vi "CSTK_Button_Icon_Example.vi"() -> ()   [LabVIEW 2015]
uses:
  Library/Button Icon/CSTK_Button_Icon.xctl
  Library/Button Icon/Private/TypeDefinitions/CSTK_Button_Icon_Properties_Color.ctl
  Library/Button Icon/Private/TypeDefinitions/CSTK_Button_Icon_Properties_BorderWidth.ctl
  Library/Button Icon/Private/TypeDefinitions/CSTK_Button_Icon_Properties_BorderStyle.ctl
  Library/Button Icon/Private/TypeDefinitions/CSTK_Button_Icon_Properties_BorderRadius.ctl
  Library/Button Icon/Private/TypeDefinitions/CSTK_Button_Icon_Properties_BoolText.ctl
  Library/Button Icon/Private/TypeDefinitions/CSTK_Button_Icon_Properties_HorizontalOffset.ctl
  Library/Button Icon/Private/TypeDefinitions/CSTK_Button_Icon_Properties_Display.ctl
  Library/Button Icon/Private/TypeDefinitions/CSTK_Button_Icon_Properties_FontStyle.ctl
  Library/Button Icon/Private/TypeDefinitions/_CSTK_Button_Icon_TextProperties_FontStyle.ctl
panel:
  in  "LOGO:显示LOGO":T1
  in  "LOGO:水平偏移":T2
  in  "布尔文本:字体样式":T3={"False"={"Font Name"="", "Size"=17, "Strikeout?"=FALSE, "Italic?"=FALSE, "Underline?"=FALSE, "Outline?"=FALSE, "Shadow?"=FALSE, "Bold?"=FALSE}, "True"={"Font Name"="", "Size"=17, "Strikeout?"=FALSE, "Italic?"=FALSE, "Underline?"=FALSE, "Outline?"=FALSE, "Shadow?"=FALSE, "Bold?"=FALSE}, "True to False"={"Font Name"="", "Size"=17, "Strikeout?"=FALSE, "Italic?"=FALSE, "Underline?"=FALSE, "Outline?"=FALSE, "Shadow?"=FALSE, "Bold?"=FALSE}, "False to True"={"Font Name"="", "Size"=17, "Strikeout?"=FALSE, "Italic?"=FALSE, "Underline?"=FALSE, "Outline?"=FALSE, "Shadow?"=FALSE, "Bold?"=FALSE}, "Hover in False"={"Font Name"="", "Size"=17, "Strikeout?"=FALSE, "Italic?"=FALSE, "Underline?"=FALSE, "Outline?"=FALSE, "Shadow?"=FALSE, "Bold?"=FALSE}, "Hover in True"={"Font Name"="", "Size"=17, "Strikeout?"=FALSE, "Italic?"=FALSE, "Underline?"=FALSE, "Outline?"=FALSE, "Shadow?"=FALSE, "Bold?"=FALSE}}
  in  "布尔文本:显示文本":T1
  in  "布尔文本:文本颜色":T5
  in  "布尔文本:水平偏移":T2
  in  "布尔文本":T6
  in  "边框颜色":T5
  in  "边框属性:圆角半径":T7
  in  "边框属性:线条样式":T8
  in  "边框属性:线条宽度":T9
  in  "背景颜色":T5
  in  "按钮大小":cluster{"Width":u32, "Height":u32}
  in  "停止VI按钮":bool
  in  "写入属性":bool
  in  "刷新属性":bool
  in  "CSTK_Button_Icon_Control":bool(xcontrol)
  out "Record":string
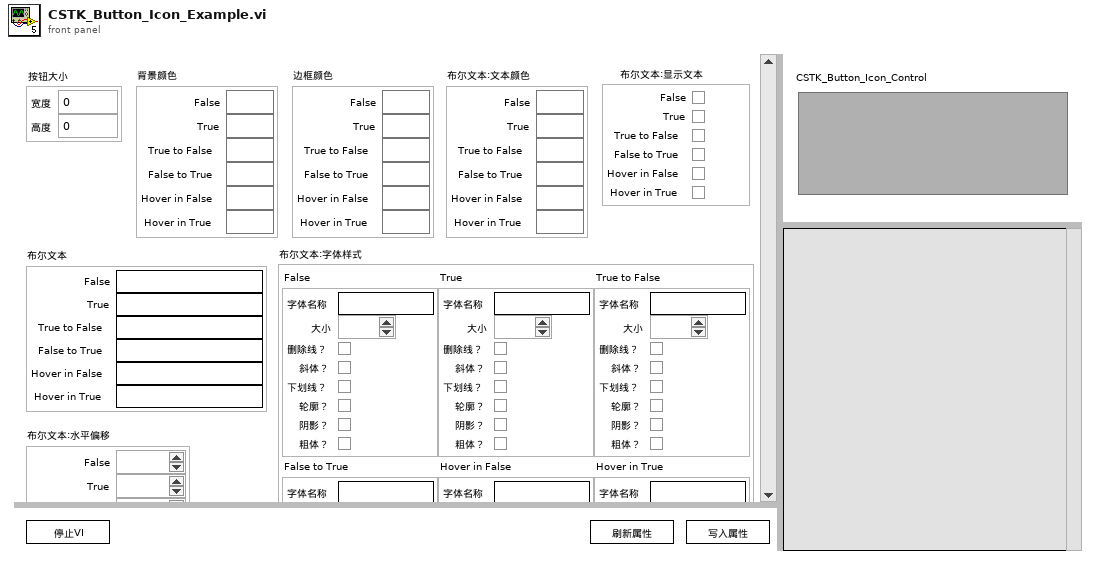
[diagram p1: front panel]
types:
  T1 = typedef "CSTK_Button_Icon.xctl/CSTK_Button_Icon_Properties_Display.ctl" = cluster{"False":bool, "True":bool, "True to False":bool, "False to True":bool, "Hover in False":bool, "Hover in True":bool}
  T2 = typedef "CSTK_Button_Icon.xctl/CSTK_Button_Icon_Properties_HorizontalOffset.ctl" = cluster{"False":i16, "True":i16, "True to False":i16, "False to True":i16, "Hover in False":i16, "Hover in True":i16}
  T3 = typedef "CSTK_Button_Icon.xctl/CSTK_Button_Icon_Properties_FontStyle.ctl" = cluster{"False":T4, "True":T4, "True to False":T4, "False to True":T4, "Hover in False":T4, "Hover in True":T4}
  T4 = typedef "CSTK_Button_Icon.xctl/_CSTK_Button_Icon_TextProperties_FontStyle.ctl" = cluster{"Font Name":string, "Size":i16, "Strikeout?":bool, "Italic?":bool, "Underline?":bool, "Outline?":bool, "Shadow?":bool, "Bold?":bool}
  T5 = typedef "CSTK_Button_Icon.xctl/CSTK_Button_Icon_Properties_Color.ctl" = cluster{"False":u32, "True":u32, "True to False":u32, "False to True":u32, "Hover in False":u32, "Hover in True":u32}
  T6 = typedef "CSTK_Button_Icon.xctl/CSTK_Button_Icon_Properties_BoolText.ctl" = cluster{"False":string, "True":string, "True to False":string, "False to True":string, "Hover in False":string, "Hover in True":string}
  T7 = typedef "CSTK_Button_Icon.xctl/CSTK_Button_Icon_Properties_BorderRadius.ctl" = cluster{"False":i16, "True":i16, "True to False":i16, "False to True":i16, "Hover in False":i16, "Hover in True":i16}
  T8 = typedef "CSTK_Button_Icon.xctl/CSTK_Button_Icon_Properties_BorderStyle.ctl" = cluster{"False":enum32{"Solid", "Dash", "Dot", "DashDot", "DashDotDot"}, "True":enum32{"Solid", "Dash", "Dot", "DashDot", "DashDotDot"}, "True to False":enum32{"Solid", "Dash", "Dot", "DashDot", "DashDotDot"}, "False to True":enum32{"Solid", "Dash", "Dot", "DashDot", "DashDotDot"}, "Hover in False":enum32{"Solid", "Dash", "Dot", "DashDot", "DashDotDot"}, "Hover in True":enum32{"Solid", "Dash", "Dot", "DashDot", "DashDotDot"}}
  T9 = typedef "CSTK_Button_Icon.xctl/CSTK_Button_Icon_Properties_BorderWidth.ctl" = cluster{"False":u16, "True":u16, "True to False":u16, "False to True":u16, "Hover in False":u16, "Hover in True":u16}
  T10 = cluster{"Action":string, "Value":variant, "Remark":string}
  T11 = cluster{"Action":string, "Value":string, "Remark":string}
  T12 = typedef "LVBoundsTypeDef.ctl" = cluster{"Width":u32, "Height":u32}
  T13 = typedef "LVRectTypeDef.ctl" = cluster{"Left":i16, "Top":i16, "Right":i16, "Bottom":i16}
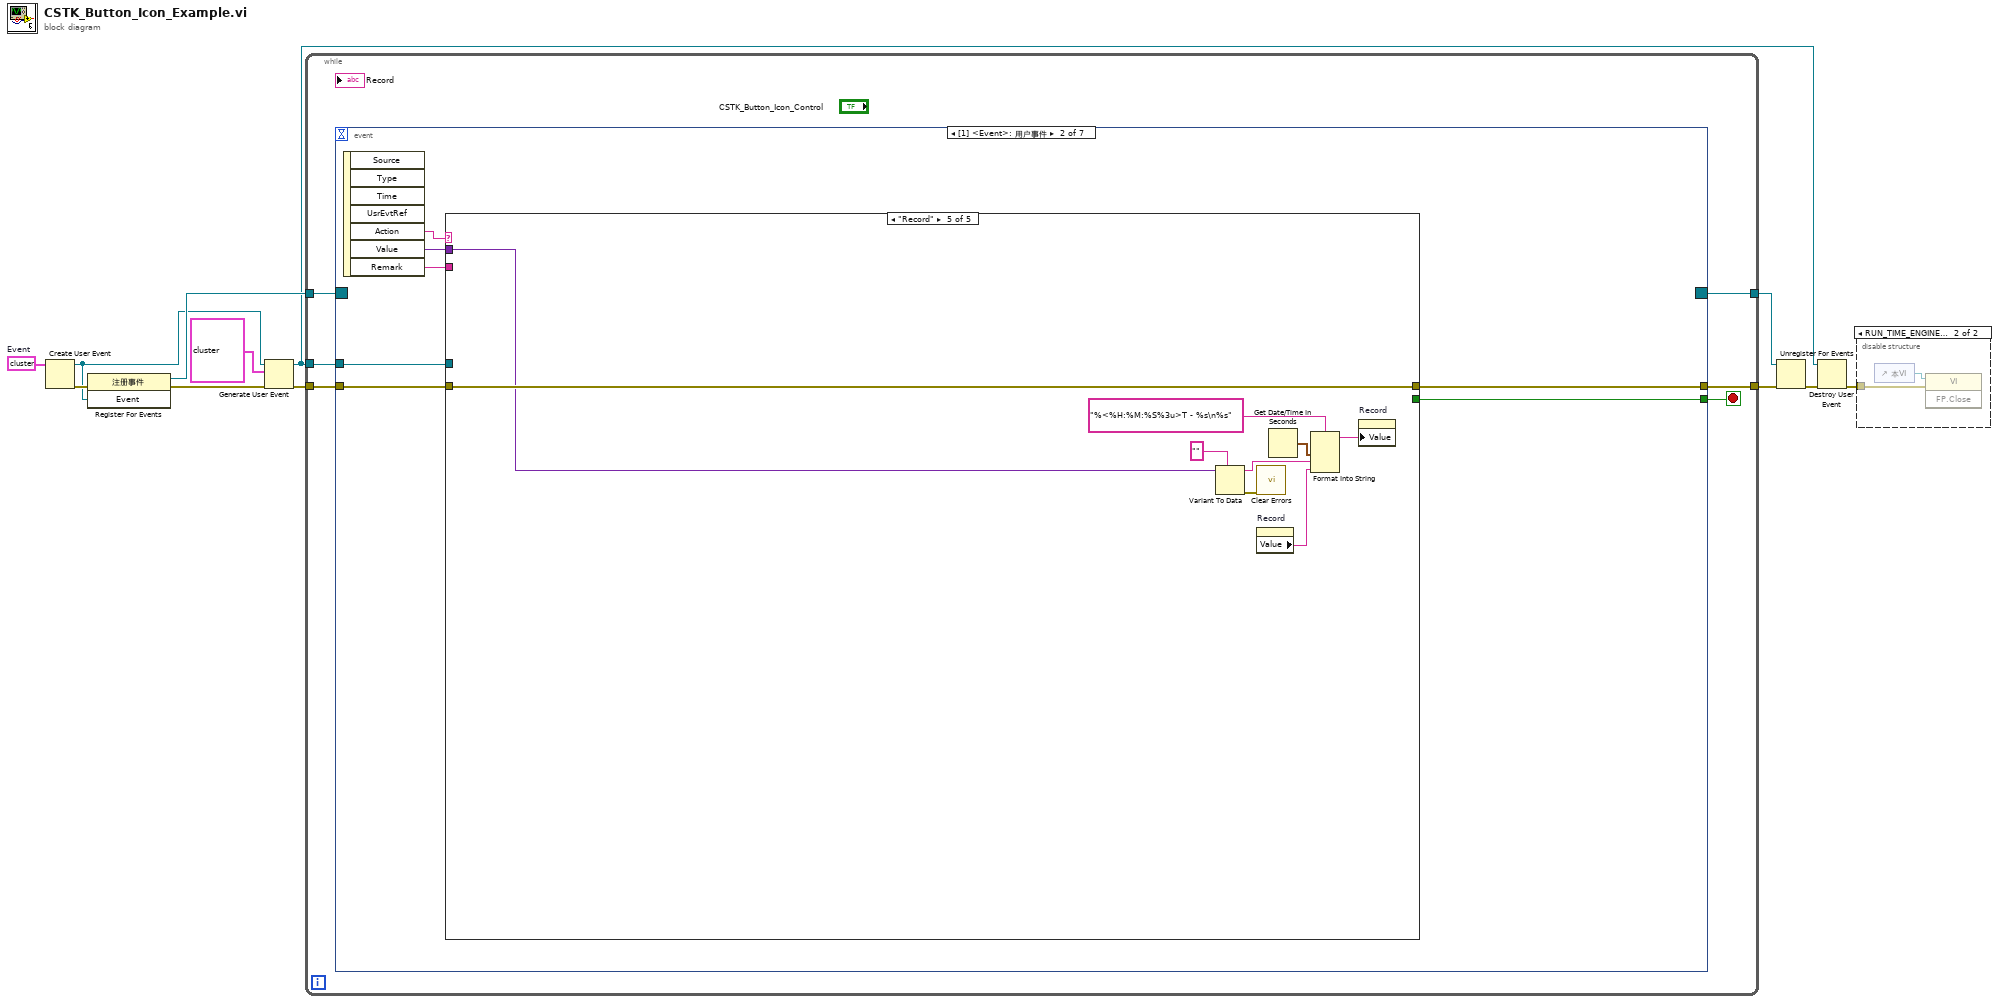
[diagram p0: block diagram]
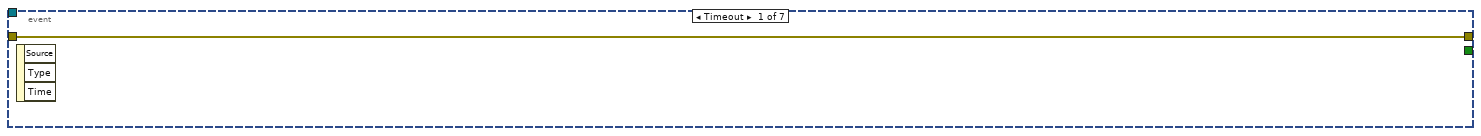
[diagram p3: hidden frame]
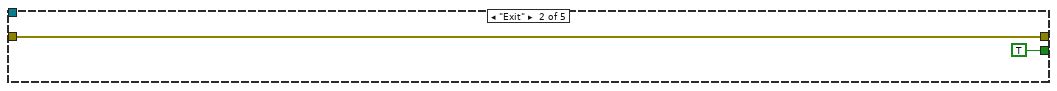
[diagram p5: hidden frame]
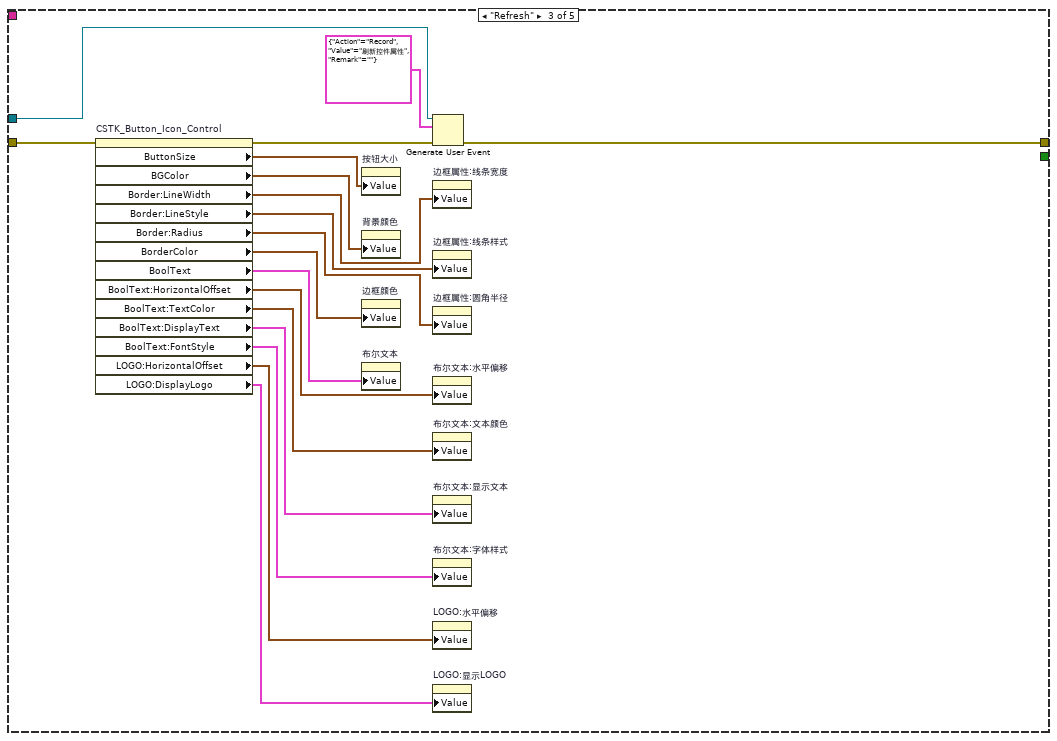
[diagram p6: hidden frame]
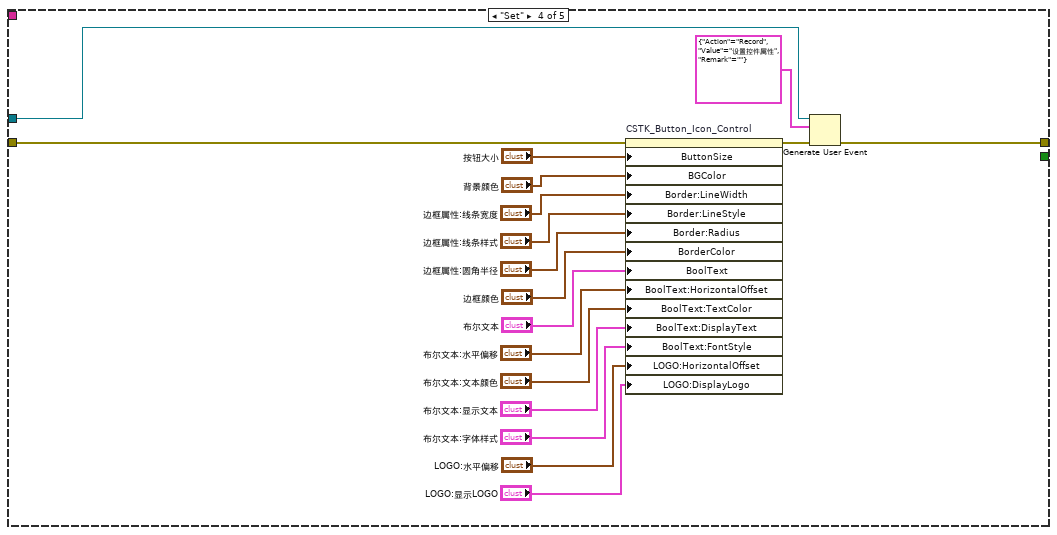
[diagram p7: hidden frame]
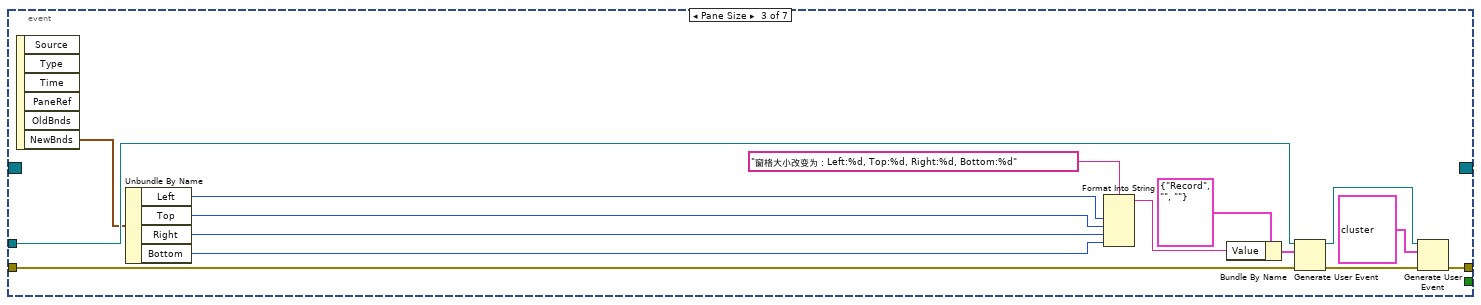
[diagram p8: hidden frame]
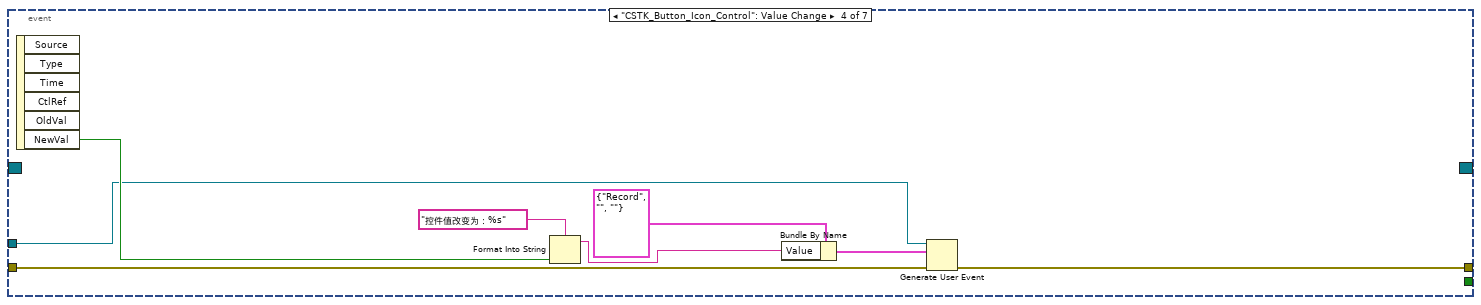
[diagram p9: hidden frame]
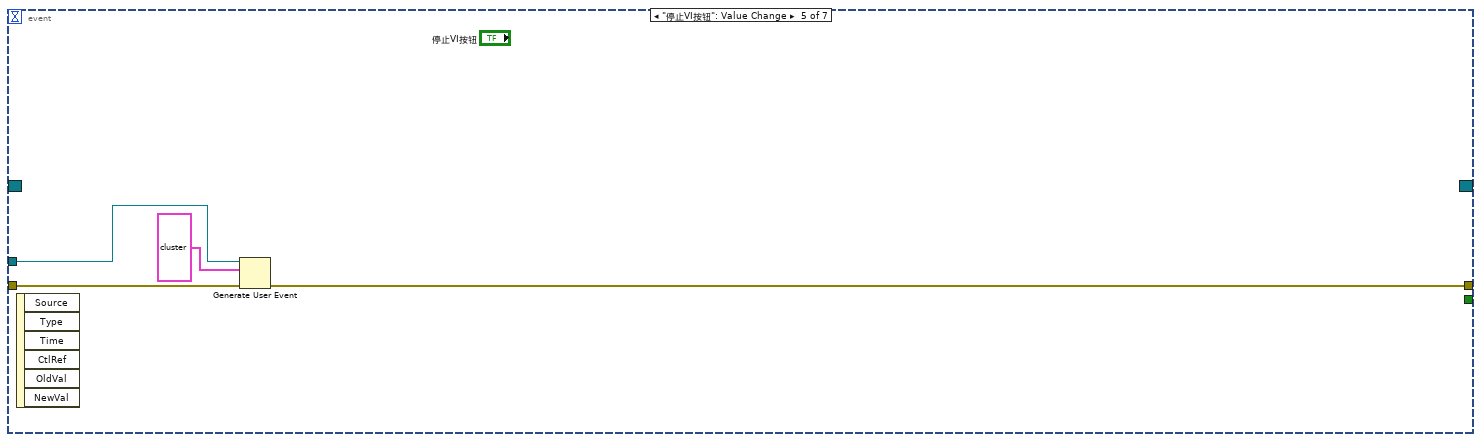
[diagram p10: hidden frame]
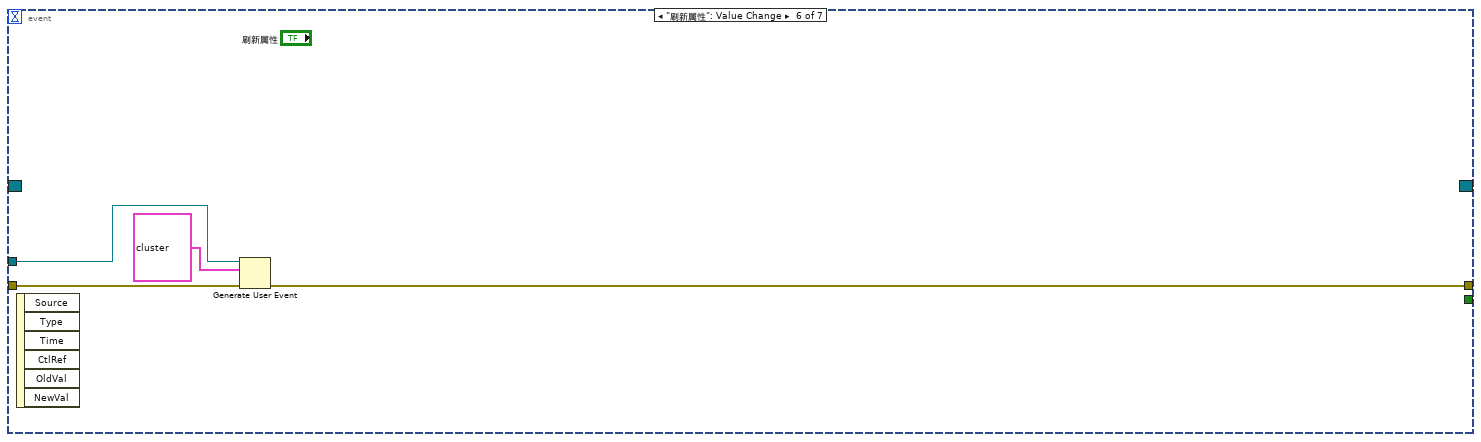
[diagram p11: hidden frame]
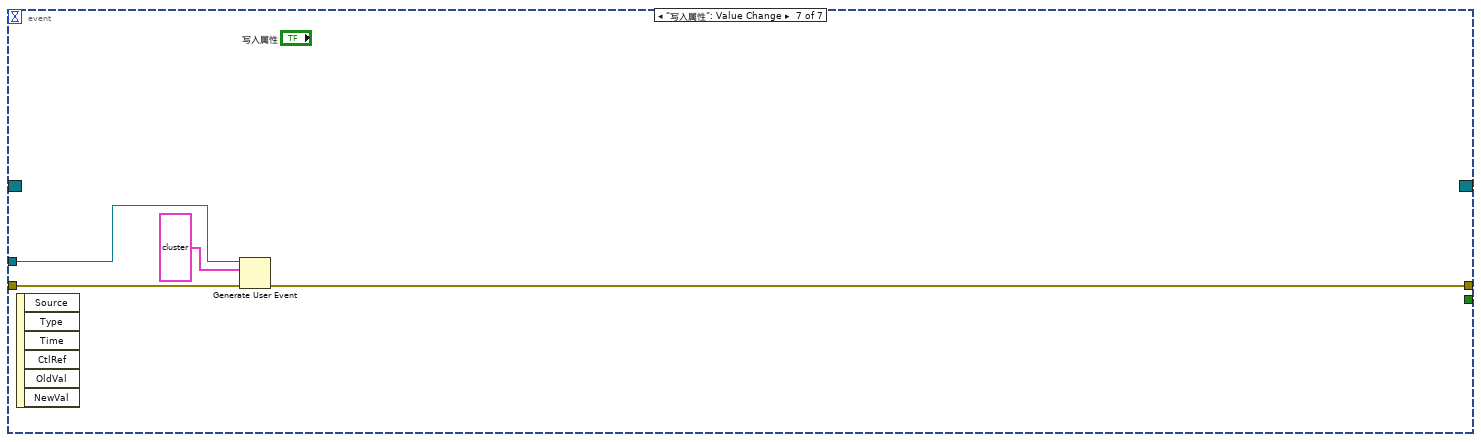
[diagram p12: hidden frame]
diagram:
  w12 = T10 {"Action"="", "Value"=variant, "Remark"=""}  # Event
  n1 = Create User Event(user event datatype=w12) -> (user event=w4:refnum<user-event>, error out=w11:errorcluster)  [unwired: 1 in]
  n2 = register-events(error in=w11, w4) -> (reference out=w10:refnum<event-registration>, error out=w6:errorcluster)  [unwired: 1 in]
  n3 = Generate User Event(user event=w4, event data cluster=T10 {"Action"="Refresh", "Value"=variant, "Remark"=""} ("事件数据"), error in=w6) -> (user event out=w2:refnum<user-event>, error out=w5:errorcluster)  [unwired: 1 in]
  n4 = while {
    tunnel: w10 -> [w18]
    tunnel: [w17] -> w9
    tunnel: w5 -> [w15]
    tunnel: [w16] -> w8
    tunnel: w2 -> [w14]
    stop <- w13 stop-if-true
    n5 = event shown="[1] <Event>: 用户事件" {
      selector: w18 -> [_ _ _ _ _ _ _]
      dyn-events: [_ _ _ _ _ _ _] -> w17
      timeout: _ -> [_ _ _ _ _ _ _]
      tunnel: [w19 w24 w75 w95 w100 w102 w107] -> w16
      tunnel: w15 -> [w19 w25 w88 w96 w101 w104 w108]
      tunnel: w14 -> [_ w20 w87 w90 w99 w103 w106]
      tunnel: [_ w21 _ _ _ _ _] -> w13
      event Timeout {
        n6 = event-data() -> ()  [unwired: 1 in, 3 out]
      }
      event User Event {
        n7 = event-data() -> ("Action"=w26:string, "Value"=w23:variant, "Remark"=w22:string)  [unwired: 1 in, 4 out]
        n8 = case shown="\"Record\"" w26 {
          tunnel: [w27 w29 w31 w49 w74] -> w24
          tunnel: w25 -> [w27 w29 w34 w65 w74]
          tunnel: w23 -> [_ _ _ _ w70]
          tunnel: w22 -> [_ _ _ _ _]
          tunnel: [_ TRUE _ _ _] -> w21
          tunnel: w20 -> [_ _ w30 w48 _]
          frame Default {
          }
          frame "Exit" {
          }
          frame "Refresh" {
            n9 = property on="CSTK_Button_Icon_Control" class="CSTK_Button_Icon (严格)"(error in=w34) -> (error out=w32:errorcluster, "ButtonSize"=w46:T12, "BGColor"=w47:T5, "Border:LineWidth"=w45:T9, "Border:LineStyle"=w44:T8, "Border:Radius"=w43:T7, "BorderColor"=w42:T5, "BoolText"=w41:T6, "BoolText:HorizontalOffset"=w40:T2, "BoolText:TextColor"=w39:T5, "BoolText:DisplayText"=w38:T1, "BoolText:FontStyle"=w37:T3, "LOGO:HorizontalOffset"=w36:T2, "LOGO:DisplayLogo"=w35:T1)  [unwired: 1 in, 1 out]
            n10 = property on="按钮大小" class="Clust (严格)"("Value"=w46) -> ()  [unwired: 2 in, 2 out]
            n11 = property on="背景颜色" class="Clust (严格)"("Value"=w47) -> ()  [unwired: 2 in, 2 out]
            n12 = property on="边框颜色" class="Clust (严格)"("Value"=w42) -> ()  [unwired: 2 in, 2 out]
            n13 = property on="布尔文本" class="Clust (严格)"("Value"=w41) -> ()  [unwired: 2 in, 2 out]
            n14 = Generate User Event(user event=w30, event data cluster=T11 {"Action"="Record", "Value"="刷新控件属性", "Remark"=""} ("事件数据"), error in=w32) -> (error out=w31:errorcluster)  [unwired: 1 in, 1 out]
            n15 = property on="边框属性:线条宽度" class="Clust (严格)"("Value"=w45) -> ()  [unwired: 2 in, 2 out]
            n16 = property on="边框属性:线条样式" class="Clust (严格)"("Value"=w44) -> ()  [unwired: 2 in, 2 out]
            n17 = property on="边框属性:圆角半径" class="Clust (严格)"("Value"=w43) -> ()  [unwired: 2 in, 2 out]
            n18 = property on="布尔文本:水平偏移" class="Clust (严格)"("Value"=w40) -> ()  [unwired: 2 in, 2 out]
            n19 = property on="布尔文本:文本颜色" class="Clust (严格)"("Value"=w39) -> ()  [unwired: 2 in, 2 out]
            n20 = property on="布尔文本:显示文本" class="Clust (严格)"("Value"=w38) -> ()  [unwired: 2 in, 2 out]
            n21 = property on="布尔文本:字体样式" class="Clust (严格)"("Value"=w37) -> ()  [unwired: 2 in, 2 out]
            n22 = property on="LOGO:水平偏移" class="Clust (严格)"("Value"=w36) -> ()  [unwired: 2 in, 2 out]
            n23 = property on="LOGO:显示LOGO" class="Clust (严格)"("Value"=w35) -> ()  [unwired: 2 in, 2 out]
          }
          frame "Set" {
            n24 = property on="CSTK_Button_Icon_Control" class="CSTK_Button_Icon (严格)"(error in=w65, "ButtonSize"="按钮大小", "BGColor"="背景颜色", "Border:LineWidth"="边框属性:线条宽度", "Border:LineStyle"="边框属性:线条样式", "Border:Radius"="边框属性:圆角半径", "BorderColor"="边框颜色", "BoolText"="布尔文本", "BoolText:HorizontalOffset"="布尔文本:水平偏移", "BoolText:TextColor"="布尔文本:文本颜色", "BoolText:DisplayText"="布尔文本:显示文本", "BoolText:FontStyle"="布尔文本:字体样式", "LOGO:HorizontalOffset"="LOGO:水平偏移", "LOGO:DisplayLogo"="LOGO:显示LOGO") -> (error out=w50:errorcluster)  [unwired: 1 in, 1 out]
            n25 = Generate User Event(user event=w48, event data cluster=T11 {"Action"="Record", "Value"="设置控件属性", "Remark"=""} ("事件数据"), error in=w50) -> (error out=w49:errorcluster)  [unwired: 1 in, 1 out]
          }
          frame "Record" {
            n26 = Variant To Data(type="", Variant=w70) -> (data=w68:string, error out=w69:errorcluster)  [unwired: 1 in]
            n27 = call <vilib>:"Clear Errors.vi"("error in (no error)"=w69) -> ()  [unwired: 5 in, 2 out]
            n28 = property on="Record" class="Str"() -> ("Value"=w67:string)  [unwired: 2 in, 2 out]
            n29 = Get Date/Time In Seconds() -> (seconds since 1Jan1904=w72:timestamp)
            n30 = Format Into String(format string="%<%H:%M:%S%3u>T - %s\n%s" ("格式字符串"), w72, w68, w67) -> (resulting string=w66:string)  [unwired: 2 in, 1 out]
            n31 = property on="Record" class="Str"("Value"=w66) -> ()  [unwired: 2 in, 2 out]
          }
        }
      }
      event Pane Size {
        n32 = event-data() -> ("NewBnds"=w84:T13)  [unwired: 1 in, 5 out]
        n33 = Unbundle By Name(w84) -> ("Left"=w83:i16, "Top"=w82:i16, "Right"=w81:i16, "Bottom"=w80:i16)
        n34 = Format Into String(format string="窗格大小改变为：Left:%d, Top:%d, Right:%d, Bottom:%d" ("格式字符串"), w83, w82, w81, w80) -> (resulting string=w79:string)  [unwired: 2 in, 1 out]
        n35 = Bundle By Name(cluster=T11 {"Action"="Record", "Value"="", "Remark"=""} ("事件数据"), "Value"=w79) -> (w86:T11)
        n36 = Generate User Event(user event=w87, event data cluster=w86, error in=w88) -> (user event out=w76:refnum<user-event>, error out=w77:errorcluster)  [unwired: 1 in]
        n37 = Generate User Event(user event=w76, event data cluster=T10 {"Action"="Refresh", "Value"=variant, "Remark"=""} ("事件数据"), error in=w77) -> (error out=w75:errorcluster)  [unwired: 1 in, 1 out]
      }
      event "CSTK_Button_Icon_Control": Value Change {
        n38 = event-data() -> ("NewVal"=w92:bool)  [unwired: 1 in, 5 out]
        n39 = Format Into String(format string="控件值改变为：%s" ("格式字符串"), w92) -> (resulting string=w91:string)  [unwired: 2 in, 1 out]
        n40 = Bundle By Name(cluster=T11 {"Action"="Record", "Value"="", "Remark"=""} ("事件数据"), "Value"=w91) -> (w94:T11)
        n41 = Generate User Event(user event=w90, event data cluster=w94, error in=w96) -> (error out=w95:errorcluster)  [unwired: 1 in, 1 out]
      }
      event "停止VI按钮": Value Change {
        n42 = event-data() -> ()  [unwired: 1 in, 6 out]
        n43 = Generate User Event(user event=w99, event data cluster=T10 {"Action"="Exit", "Value"=variant, "Remark"=""} ("事件数据"), error in=w101) -> (error out=w100:errorcluster)  [unwired: 1 in, 1 out]
      }
      event "刷新属性": Value Change {
        n44 = event-data() -> ()  [unwired: 1 in, 6 out]
        n45 = Generate User Event(user event=w103, event data cluster=T10 {"Action"="Refresh", "Value"=variant, "Remark"=""} ("事件数据"), error in=w104) -> (error out=w102:errorcluster)  [unwired: 1 in, 1 out]
      }
      event "写入属性": Value Change {
        n46 = event-data() -> ()  [unwired: 1 in, 6 out]
        n47 = Generate User Event(user event=w106, event data cluster=T10 {"Action"="Set", "Value"=variant, "Remark"=""} ("事件数据"), error in=w108) -> (error out=w107:errorcluster)  [unwired: 1 in, 1 out]
      }
    }
  }
  n48 = Unregister For Events(event registration refnum=w9, error in=w8) -> (error out=w7:errorcluster)
  n49 = Destroy User Event(user event=w2, error in=w7) -> (error out=w1:errorcluster)
  n50 = disable-structure shown="RUN_TIME_ENGINE==True" {
    disable-tunnel: w1 -> [_ w111]
    frame condition #0 (active) {
    }
    frame condition #1 {
      n51 = control-ref of="本VI"() -> (w110:refnum<vi>)
      n52 = invoke class="VI" method="FP.Close"(reference=w110, error in=w111) -> ()  [unwired: 1 in, 3 out]
    }
  }
